vi "offset_waveform_bundle.vi"(1 "Offset":dbl format="%#_13g", 3 "Bundled Waveform Data":T1) -> (0 "Offseted Waveform Bundle":T1)   [LabVIEW 2019]
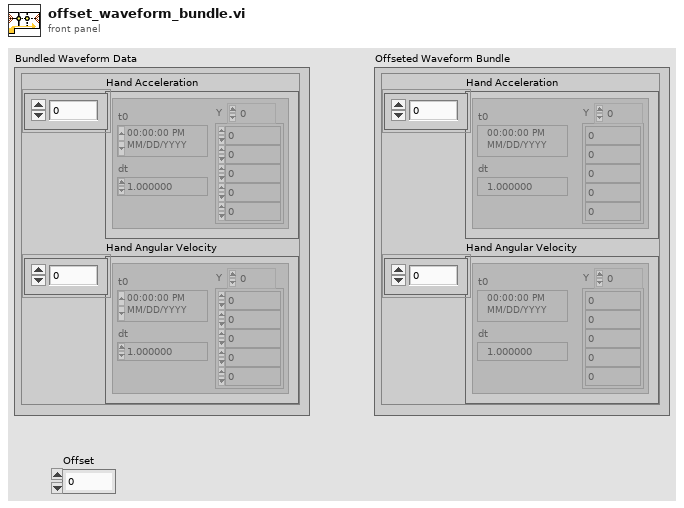
[diagram p1: front panel]
types:
  T1 = cluster{"Hand Acceleration":waveform(dbl)[], "Hand Angular Velocity":waveform(dbl)[]}
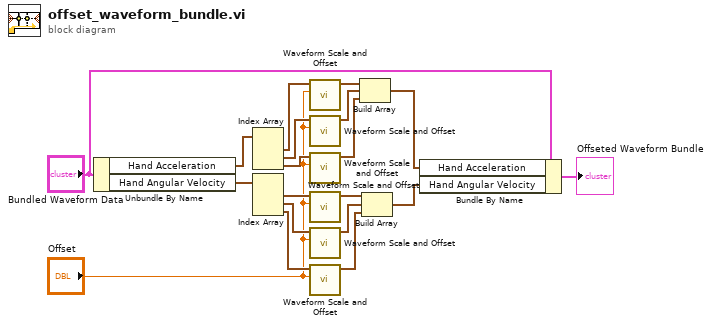
[diagram p0: block diagram]
diagram:
  n1 = Unbundle By Name("Bundled Waveform Data") -> ("Hand Acceleration"=w19:waveform(dbl)[], "Hand Angular Velocity"=w18:waveform(dbl)[])
  n2 = Index Array(array=w19) -> (element #1=w17:waveform(dbl), element #2=w16:waveform(dbl), element #3=w15:waveform(dbl))  [unwired: 3 in]
  n3 = Index Array(array=w18) -> (element #1=w14:waveform(dbl), element #2=w13:waveform(dbl), element #3=w12:waveform(dbl))  [unwired: 3 in]
  n4 = call <vilib>:"Waveform Scale and Offset.vi"("offset"="Offset", "waveform in"=w17) -> ("waveform out"=w9:waveform(dbl))  [unwired: 8 in, 1 out]
  n5 = call <vilib>:"Waveform Scale and Offset.vi"("offset"="Offset", "waveform in"=w16) -> ("waveform out"=w8:waveform(dbl))  [unwired: 8 in, 1 out]
  n6 = call <vilib>:"Waveform Scale and Offset.vi"("offset"="Offset", "waveform in"=w15) -> ("waveform out"=w7:waveform(dbl))  [unwired: 8 in, 1 out]
  n7 = call <vilib>:"Waveform Scale and Offset.vi"("offset"="Offset", "waveform in"=w14) -> ("waveform out"=w10:waveform(dbl))  [unwired: 8 in, 1 out]
  n8 = call <vilib>:"Waveform Scale and Offset.vi"("offset"="Offset", "waveform in"=w13) -> ("waveform out"=w6:waveform(dbl))  [unwired: 8 in, 1 out]
  n9 = call <vilib>:"Waveform Scale and Offset.vi"("offset"="Offset", "waveform in"=w12) -> ("waveform out"=w5:waveform(dbl))  [unwired: 8 in, 1 out]
  n10 = Build Array(w9, w8, w7) -> (w3:waveform(dbl)[])
  n11 = Build Array(w10, w6, w5) -> (w2:waveform(dbl)[])
  n12 = Bundle By Name(cluster="Bundled Waveform Data", "Hand Acceleration"=w3, "Hand Angular Velocity"=w2) -> (→"Offseted Waveform Bundle":T1)
